vi "Get Graph.vi"(0 "Data3D in":refnum<class "Data3D.lvclass">, 11 "error in (no error)":errorcluster) -> (4 "Data3D out":refnum<class "Data3D.lvclass">, 6 "X":dbl[](array[numeric]), 8 "Y":dbl[](array[numeric]), 10 "Z matrix":dbl[][](array[numeric]), 15 "error out":errorcluster)   [LabVIEW 2014, in "Data3D.lvclass"]
uses:
  Data3D.lvclass
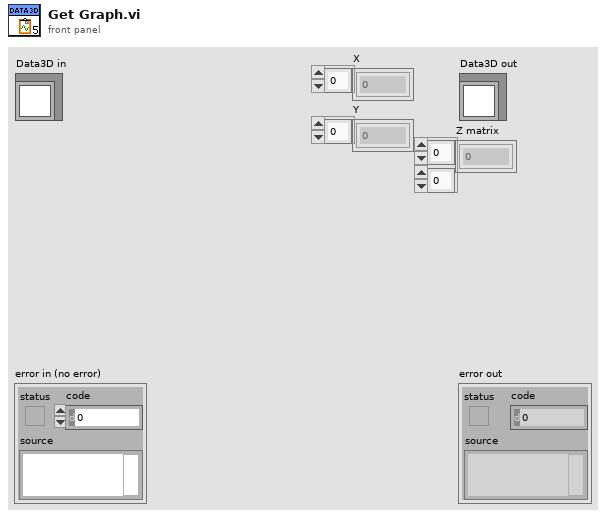
[diagram p1: front panel]
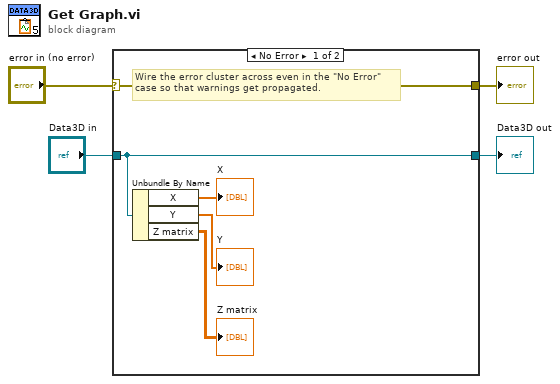
[diagram p0: block diagram]
diagram:
  n1 = case shown="No Error" "error in (no error)" {
    selector: "error in (no error)" -> [w9 w11]
    tunnel: [w9 w11] -> w3
    tunnel: [w8 w10] -> w1
    tunnel: "Data3D in" -> [w8 w10]
    frame No Error {
      # "Wire the error cluster across even in the \"No Error\"\ncase so that warnings get propagated."
      n2 = Unbundle By Name(w8) -> ("X"=→"X":dbl[], "Y"=→"Y":dbl[], "Z matrix"=→"Z matrix":dbl[][])
    }
    frame Error {
    }
  }
  "error out" <- w3
  "Data3D out" <- w1
